vi "Base_projet_meteo.vi"() -> ()   [LabVIEW 2014]
uses:
  <vilib>/Instr/_visa.llb/VISA Configure Serial Port (Instr).vi
panel:
  out "temperature":fxp<+/-,64,32>
  out "temperature":dbl(graph)
  in  "Humidity":string(combo)
  in  "Pressure":string(combo)
  out "Humidity":dbl(graph)
  out "Pressure":dbl(graph)
  in  "?":bool
  in  "Boolean 2":bool
  in  "Boolean":bool
  in  "temperature":string(combo)
  in  "Humidity":dbl=5.0 min=5.0 step=1.0
  in  "Pressure":dbl=5.0 min=5.0 step=1.0
  in  "temperature":dbl=5.0 min=5.0 step=1.0
  out "Humidity":fxp<+/-,64,32>
  out "Pressure":fxp<+/-,64,32>
  out "Lecture sur le port SERIE":string
  in  "?":bool
  in  "VISA resource name":refnum<visa-resource-name> caption="Choix du port de COM"
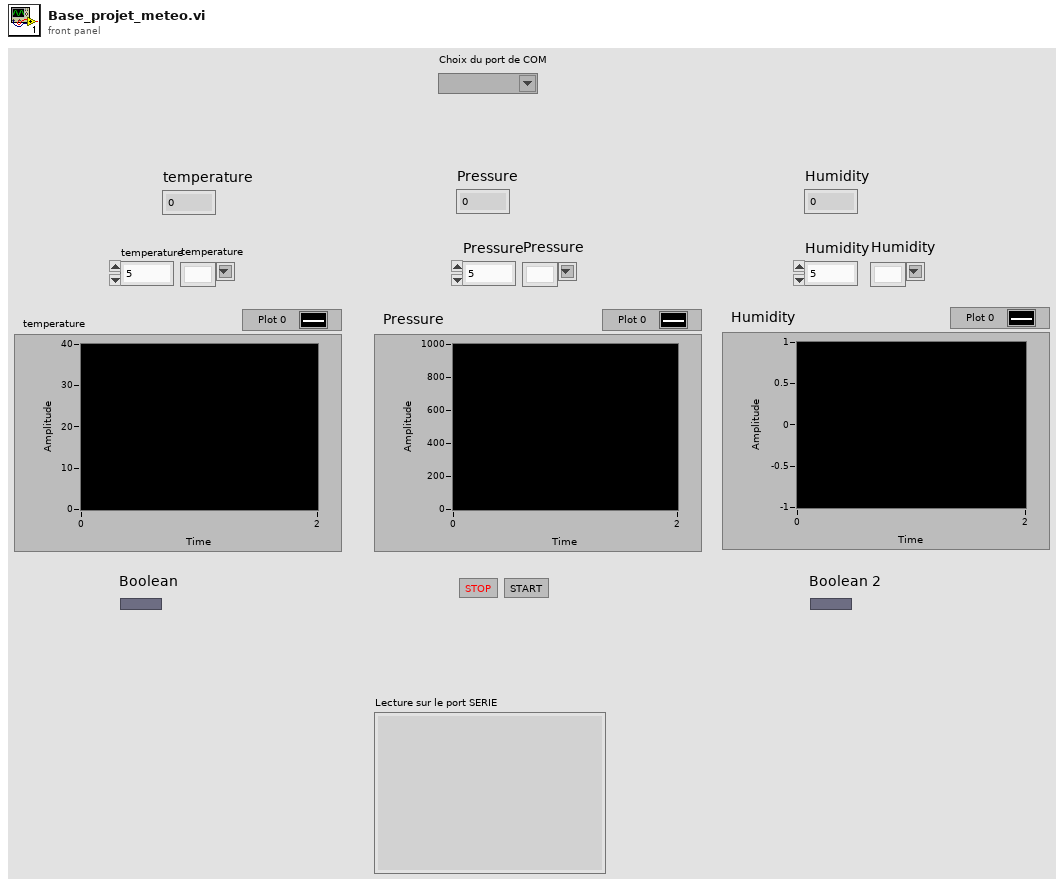
[diagram p1: front panel]
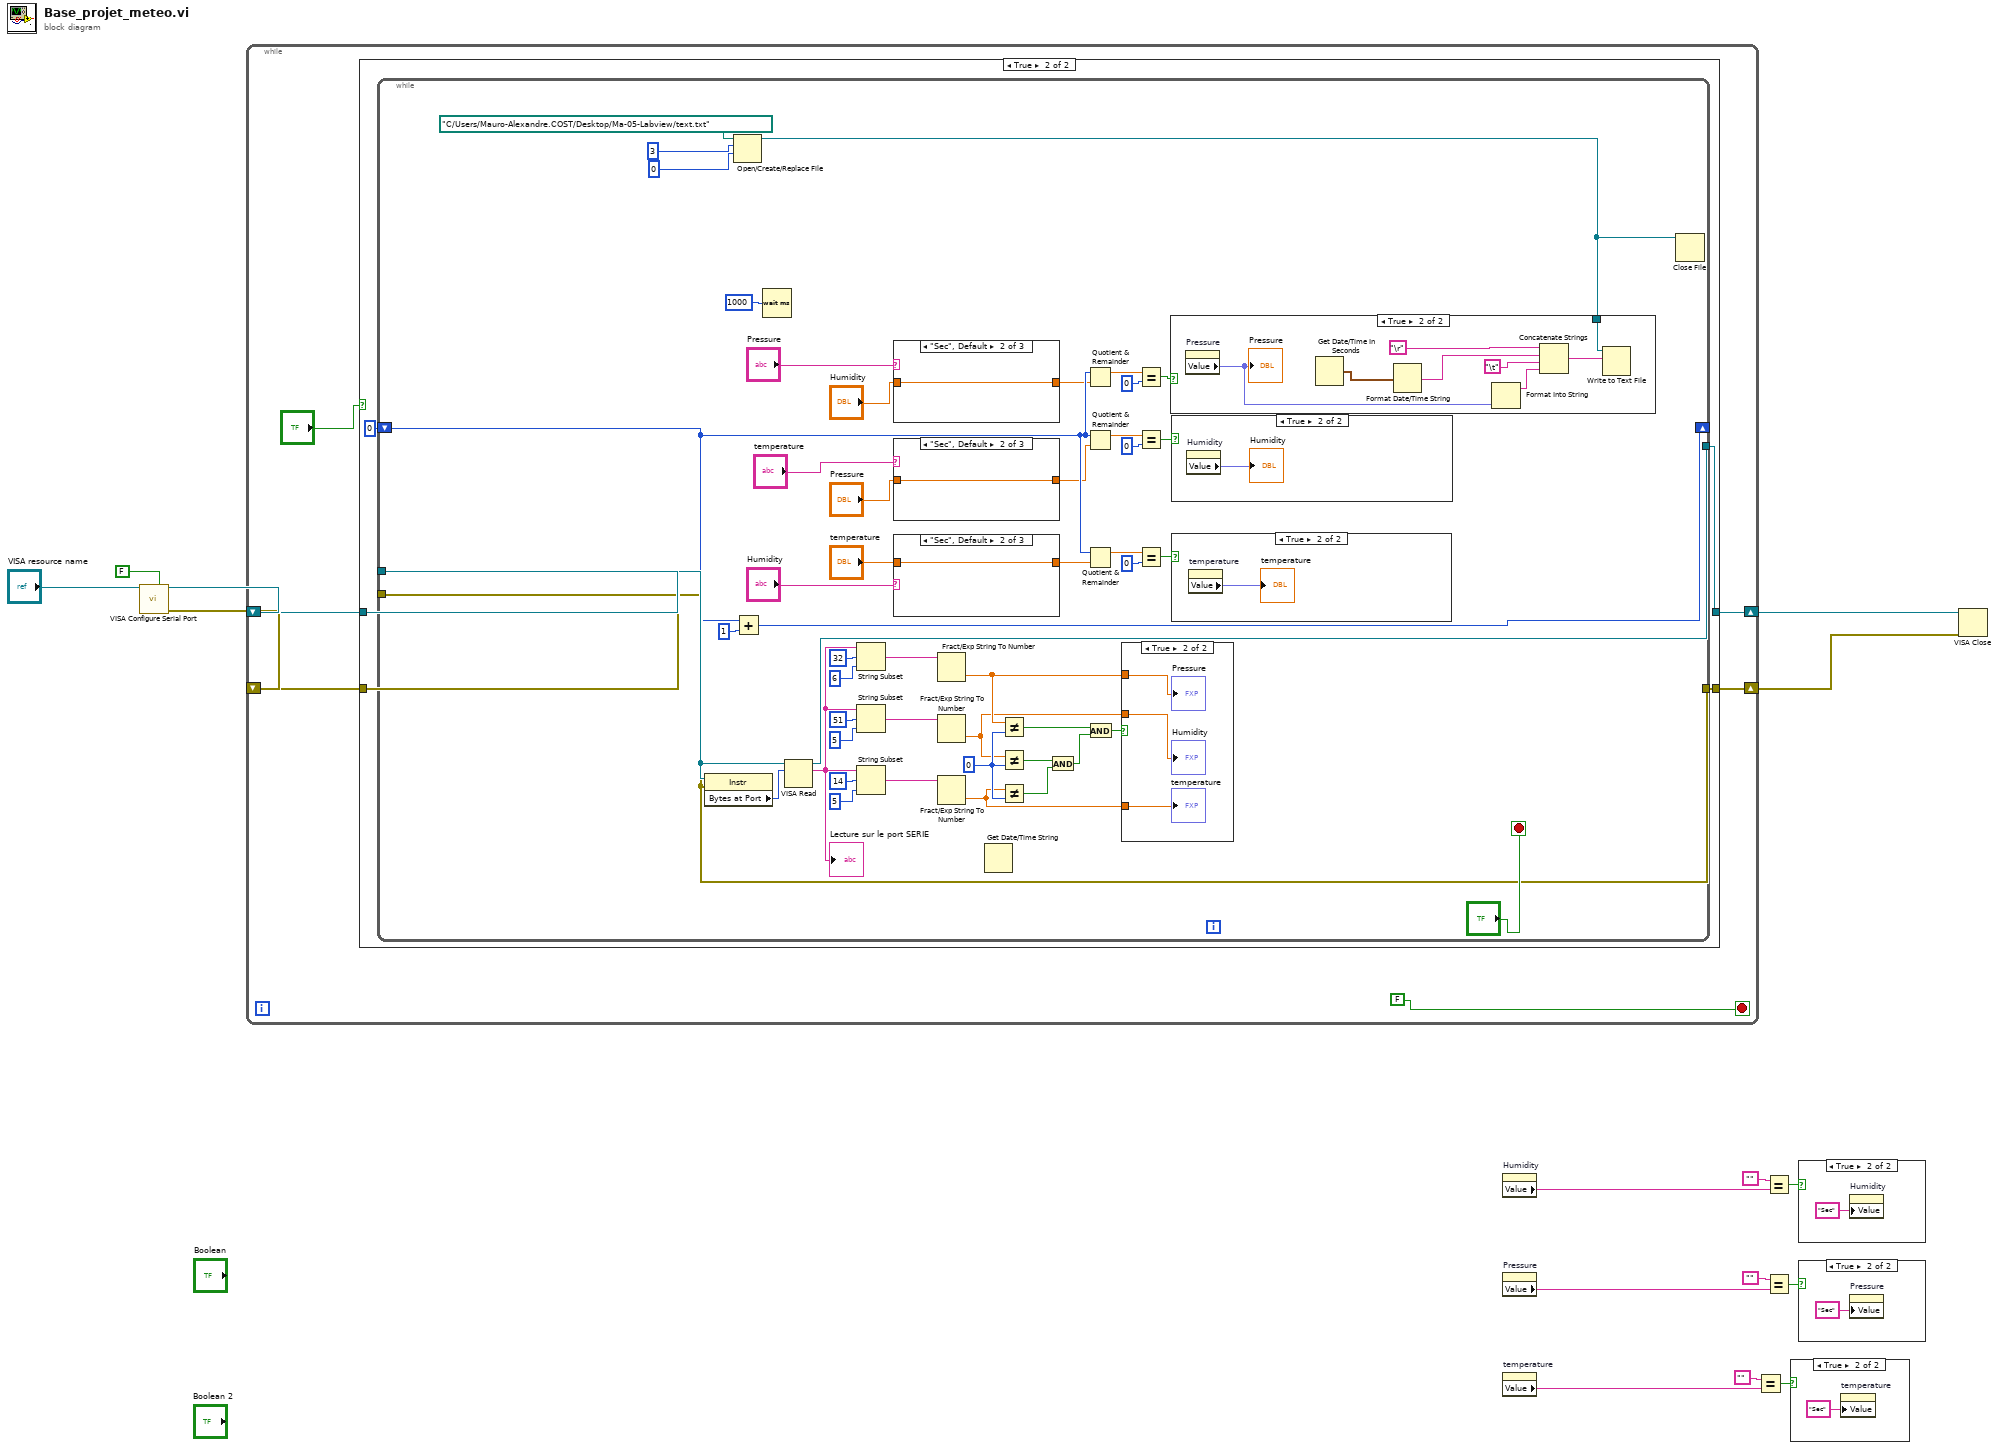
[diagram p0: block diagram]
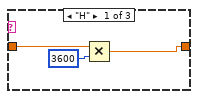
[diagram p3: hidden frame]
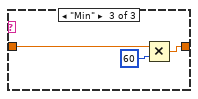
[diagram p4: hidden frame]
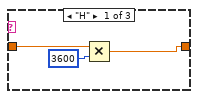
[diagram p5: hidden frame]
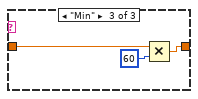
[diagram p6: hidden frame]
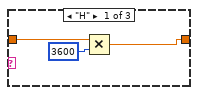
[diagram p7: hidden frame]
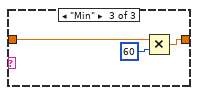
[diagram p8: hidden frame]
diagram:
  n1 = call-poly "VISA Configure Serial Port"("VISA resource name"="VISA resource name", "Enable Termination\nChar (T)"=FALSE ("Enable Termination\nChar (T)")) -> ("VISA resource name out"=w14:refnum<visa-resource-name>, "error out"=w12:errorcluster)  [unwired: 12 in]
  n2 = while {
    shift-right: [w18] -> w10
    shift-left: w14 -> [w21]
    shift-right: [w19] -> w11
    shift-left: w12 -> [w20]
    stop <- FALSE ("Enable Termination\nChar (T)") stop-if-true
    n3 = case shown="True" "?" {
      tunnel: w21 -> [w23 w28]
      tunnel: w20 -> [w22 w27]
      tunnel: [w22 w26] -> w19
      tunnel: [w23 w25] -> w18
      frame False {
      }
      frame True {
        n4 = while {
          tunnel: w28 -> [w76]
          tunnel: w27 -> [w74]
          tunnel: [w74] -> w26
          tunnel: [w75] -> w25
          shift-right: [w53] -> _
          shift-left: 0 -> [w43]
          stop <- "?" stop-if-true
          w50 = 0
          n5 = property class="Instr"(reference=w76, error in=w74) -> ("Bytes at Port"=w77:u32)  [unwired: 2 out]
          n6 = Open/Create/Replace File(file path (use dialog)=path "C:/Users/Mauro-Alexandre.COST/Desktop/Ma-05-Labview/text.txt", operation (0:open)=3, access (0:read/write)=0) -> (refnum out=w33:refnum<file>)  [unwired: 3 in, 2 out]
          n7 = Add(x=w43, y=1) -> (x+y=w53:i32)
          n8 = Wait (ms)(milliseconds to wait=1000) -> ()  [unwired: 1 out]
          n9 = VISA Read(VISA resource name=w76, byte count=w77) -> (VISA resource name out=w75:refnum<visa-resource-name>, read buffer=w61:string)  [unwired: 1 in, 2 out]
          "Lecture sur le port SERIE" <- w61
          n10 = String Subset(string=w61, offset (0)=32, length (rest)=6) -> (substring=w32:string)
          n11 = String Subset(string=w61, offset (0)=51, length (rest)=5) -> (substring=w69:string)
          n12 = String Subset(string=w61, offset (0)=14, length (rest)=5) -> (substring=w64:string)
          n13 = case shown="\"Sec\", Default" "Pressure" {
            tunnel: "Humidity" -> [w79 w82 w85]
            tunnel: [w80 w82 w83] -> w35
            frame "H" {
              n14 = Multiply(x=w79, y=3600) -> (x*y=w80:dbl)
            }
            frame "Sec", Default {
            }
            frame "Min" {
              n15 = Multiply(x=w85, y=60) -> (x*y=w83:dbl)
            }
          }
          n16 = case shown="\"Sec\", Default" "temperature" {
            tunnel: "Pressure" -> [w86 w89 w92]
            tunnel: [w87 w89 w90] -> w37
            frame "H" {
              n17 = Multiply(x=w86, y=3600) -> (x*y=w87:dbl)
            }
            frame "Sec", Default {
            }
            frame "Min" {
              n18 = Multiply(x=w92, y=60) -> (x*y=w90:dbl)
            }
          }
          n19 = case shown="\"Sec\", Default" "Humidity" {
            tunnel: "temperature" -> [w93 w96 w99]
            tunnel: [w94 w96 w97] -> w40
            frame "H" {
              n20 = Multiply(x=w93, y=3600) -> (x*y=w94:dbl)
            }
            frame "Sec", Default {
            }
            frame "Min" {
              n21 = Multiply(x=w99, y=60) -> (x*y=w97:dbl)
            }
          }
          n22 = Fract/Exp String To Number(string=w32) -> (number=w46:dbl)  [unwired: 3 in, 1 out]
          n23 = Fract/Exp String To Number(string=w69) -> (number=w45:dbl)  [unwired: 3 in, 1 out]
          n24 = Fract/Exp String To Number(string=w64) -> (number=w44:dbl)  [unwired: 3 in, 1 out]
          n25 = Get Date/Time String() -> ()  [unwired: 3 in, 2 out]
          n26 = Not Equal?(x=w46, y=w50) -> (x != y?=w47:bool)
          n27 = Not Equal?(x=w45, y=w50) -> (x != y?=w48:bool)
          n28 = Not Equal?(x=w44, y=w50) -> (x != y?=w49:bool)
          n29 = And(x=w48, y=w49) -> (x .and. y?=w51:bool)
          n30 = Quotient & Remainder(x=w43, y=w35) -> (x-y*floor(x/y)=w56:dbl)  [unwired: 1 out]
          n31 = Quotient & Remainder(x=w43, y=w37) -> (x-y*floor(x/y)=w59:dbl)  [unwired: 1 out]
          n32 = Quotient & Remainder(x=w43, y=w40) -> (x-y*floor(x/y)=w68:dbl)  [unwired: 1 out]
          n33 = And(x=w47, y=w51) -> (x .and. y?=w52:bool)
          n34 = case shown="True" w52 {
            tunnel: w46 -> [_ w102]
            tunnel: w45 -> [_ w101]
            tunnel: w44 -> [_ w100]
            frame False {
            }
            frame True {
              "Pressure" <- w102
              "Humidity" <- w101
              "temperature" <- w100
            }
          }
          n35 = Equal?(x=w56, y=0) -> (x = y?=w54:bool)
          n36 = Equal?(x=w59, y=0) -> (x = y?=w57:bool)
          n37 = Equal?(x=w68, y=0) -> (x = y?=w66:bool)
          n38 = case shown="True" w54 {
            tunnel: w33 -> [_ w105]
            frame False {
            }
            frame True {
              n39 = property on="Pressure" class="DigNum (strict)"() -> ("Value"=w103:fxp<+/-,64,32>)  [unwired: 2 in, 2 out]
              "Pressure" <- w103
              n40 = Get Date/Time In Seconds() -> (seconds since 1Jan1904=w108:timestamp)
              n41 = Format Date/Time String(seconds (now)=w108) -> (date/time string=w109:string)  [unwired: 2 in]
              n42 = Format Into String(w103) -> (resulting string=w104:string)  [unwired: 3 in, 1 out]
              n43 = Concatenate Strings("\r", w109, "\t", w104) -> (w106:string)
              n44 = Write to Text File(file (use dialog)=w105, text=w106) -> ()  [unwired: 2 in, 3 out]
            }
          }
          n45 = case shown="True" w57 {
            frame False {
            }
            frame True {
              n46 = property on="Humidity" class="DigNum (strict)"() -> ("Value"=→"Humidity":fxp<+/-,64,32>)  [unwired: 2 in, 2 out]
            }
          }
          n47 = case shown="True" w66 {
            frame False {
            }
            frame True {
              n48 = property on="temperature" class="DigNum (strict)"() -> ("Value"=→"temperature":fxp<+/-,64,32>)  [unwired: 2 in, 2 out]
            }
          }
          n49 = Close File(refnum=w33) -> ()  [unwired: 1 in, 2 out]
        }
      }
    }
  }
  n50 = property on="Humidity" class="CmbBox"() -> ("Value"=w9:string)  [unwired: 2 in, 2 out]
  n51 = property on="Pressure" class="CmbBox"() -> ("Value"=w4:string)  [unwired: 2 in, 2 out]
  n52 = property on="temperature" class="CmbBox"() -> ("Value"=w1:string)  [unwired: 2 in, 2 out]
  n53 = Equal?(x="", y=w1) -> (x = y?=w2:bool)
  n54 = Equal?(x="", y=w9) -> (x = y?=w7:bool)
  n55 = Equal?(x="", y=w4) -> (x = y?=w5:bool)
  n56 = case shown="True" w2 {
    frame False {
    }
    frame True {
      n57 = property on="temperature" class="CmbBox"("Value"="Sec") -> ()  [unwired: 2 in, 2 out]
    }
  }
  n58 = case shown="True" w7 {
    frame False {
    }
    frame True {
      n59 = property on="Humidity" class="CmbBox"("Value"="Sec") -> ()  [unwired: 2 in, 2 out]
    }
  }
  n60 = case shown="True" w5 {
    frame False {
    }
    frame True {
      n61 = property on="Pressure" class="CmbBox"("Value"="Sec") -> ()  [unwired: 2 in, 2 out]
    }
  }
  n62 = VISA Close(VISA resource name=w10, error in (no error)=w11) -> ()  [unwired: 1 out]
